vi "Read XML_000.vi"(8 "error in (no error)":errorcluster, 10 "XML Configuration File Path":path=path "E:/Ballard - Arinc-429 CD/Example Database/Ballard/XML_000.XML", 11 "XML Schema File Path":path=path "E:/Ballard - Arinc-429 CD/Source/System Explorer/SubVIs/Parse XML Ballard/BTI.XSD") -> (0 "error IO":errorcluster, 3 "channels":T1 {"speed" items=["Auto", "Low", "High"]; "Labels"."scheduleBuildUnit" items=["Millisecond", "Microsecond"]})   [LabVIEW 2016, in "Ballard Arinc-429 System Explorer.lvlib"]
uses:
  Ballard Arinc-429 System Explorer.lvlib
  Controls/Ballard_Channel Array.ctl
  Controls/Ballard_Channel.ctl
  Controls/Ballard_Label.ctl
  Controls/Ballard_Word.ctl
  Controls/ARINCParam.ctl
  Shared/Controls and Global/TransferType.ctl
  Controls/Channel_direction.ctl
  Controls/Channel Speed.ctl
  E:/Ballard - Arinc-429 CD/Source/System Explorer/SubVIs/Parse XML Ballard/Ballard_BTI_XML_Deserializer.dll
  Ballard_BTI_XML_Deserializer.dll
  Shared/Ballard Arinc-429 Shared.lvlib
panel:
  out "name":string
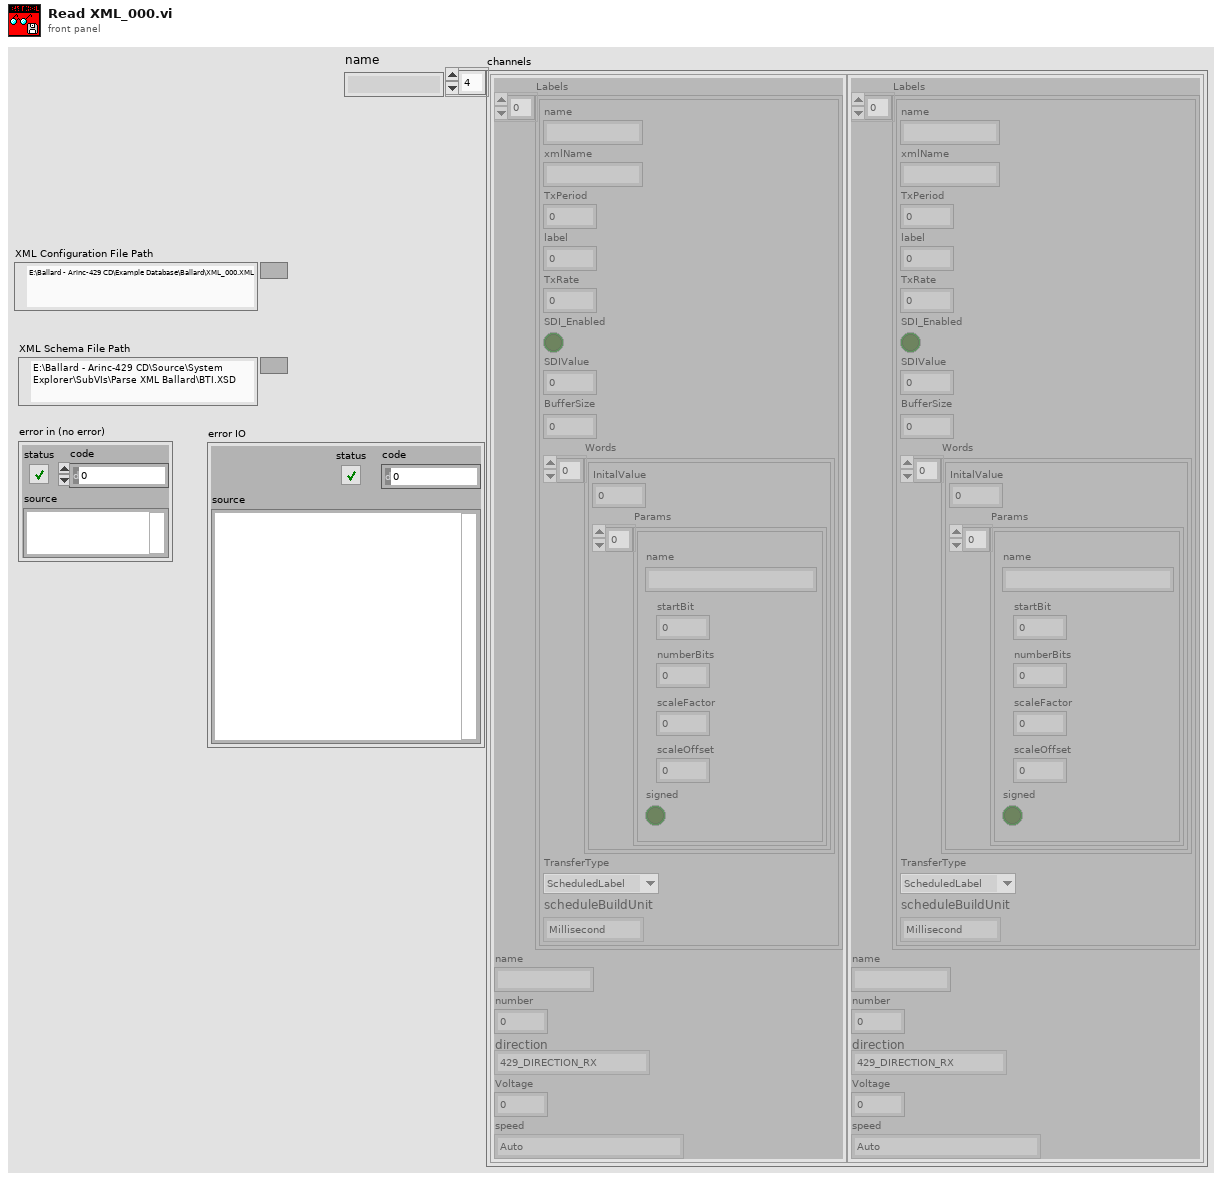
[diagram p1: front panel]
types:
  T1 = typedef "Ballard Arinc-429 System Explorer.lvlib/Ballard_Channel Array.ctl" = T2[]
  T2 = typedef "Ballard Arinc-429 System Explorer.lvlib/Ballard_Channel.ctl" = cluster{"Labels":T3[], "name":string, "number":u8, "direction":T7, "Voltage":dbl, "speed":T8}
  T3 = typedef "Ballard Arinc-429 System Explorer.lvlib/Ballard_Label.ctl" = cluster{"name":string, "xmlName":string, "TxPeriod":u32, "label":u32, "TxRate":dbl, "SDI_Enabled":bool, "SDIValue":u8, "BufferSize":u32, "Words":T4[], "TransferType":T6, "scheduleBuildUnit":i32}
  T4 = typedef "Ballard Arinc-429 System Explorer.lvlib/Ballard_Word.ctl" = cluster{"InitalValue":u32, "Params":T5[]}
  T5 = typedef "Ballard Arinc-429 System Explorer.lvlib/ARINCParam.ctl" = cluster{"name":string, "startBit":i32, "numberBits":i32, "scaleFactor":dbl, "scaleOffset":dbl, "signed":bool}
  T6 = typedef "Ballard Arinc-429 Shared.lvlib/TransferType.ctl" = enum16{"ScheduledLabel", "Acyclic", "Block", "Strobe"}
  T7 = typedef "Ballard Arinc-429 System Explorer.lvlib/Channel_direction.ctl" = enum16{"429_DIRECTION_RX", "429_DIRECTION_TX"}
  T8 = typedef "Ballard Arinc-429 System Explorer.lvlib/Channel Speed.ctl" = i32
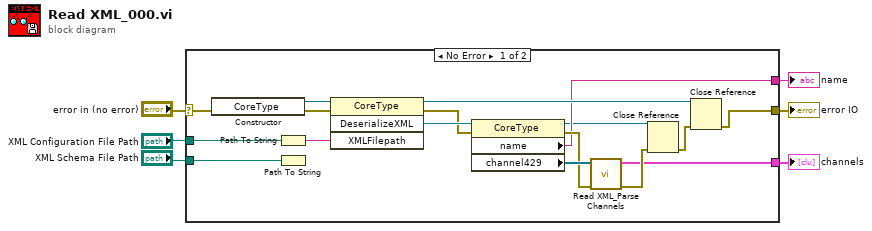
[diagram p0: block diagram]
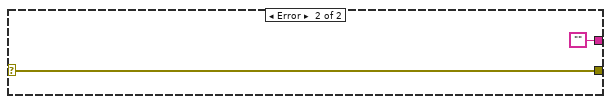
[diagram p2: hidden frame]
diagram:
  n1 = case shown="No Error" "error in (no error)" {
    selector: "error in (no error)" -> [w10 w25]
    tunnel: "XML Configuration File Path" -> [w22 _]
    tunnel: "XML Schema File Path" -> [w17 _]
    tunnel: [w12 w25] -> w3
    tunnel: [w9 _] -> w2
    tunnel: [w8 "" ("name")] -> w1
    frame No Error {
      n2 = constructor class="CoreType"(error in=w10) -> (reference out=w16:refnum<k24>, error out=w15:errorcluster)  [unwired: 2 in, 1 out]
      n3 = Path To String(path=w22) -> (string=w23:string)
      n4 = Path To String(path=w17) -> ()  [unwired: 1 out]
      n5 = invoke class="CoreType" method="DeserializeXML"(reference=w16, error in=w15, "XMLFilepath"=w23) -> (reference out=w11:refnum<k24>, error out=w20:errorcluster, "DeserializeXML"=w21:refnum<k24>)  [unwired: 1 in, 1 out]
      n6 = property class="CoreType"(reference=w21, error in=w20) -> (reference out=w7:refnum<k24>, error out=w18:errorcluster, "name"=w8:string, "channel429"=w19:refnum<k24>[])
      n7 = call "Read XML_Parse Channels.vi"("error in (no error)"=w18, "channel429"=w19) -> ("error out"=w14:errorcluster, "Array"=w9:T2[])  [unwired: 8 in]
      n8 = Close Reference(reference=w7, error in (no error)=w14) -> (error out=w13:errorcluster)
      n9 = Close Reference(reference=w11, error in (no error)=w13) -> (error out=w12:errorcluster)
    }
    frame Error {
    }
  }
  "channels" <- w2
  "error IO" <- w3
  "name" <- w1
